vi "Action.vi"(7 "Assert Message":T1, 8 "error in (no error)":errorcluster, 11 "Pause Application in":refnum<class "Pause Application.lvclass">) -> (0 "error out":errorcluster)   [LabVIEW 2016, in "Assert API Components.lvlib" / "Log Assert Core.lvlib" / "Pause Application.lvclass"]
doc: "Dynamic dispatch vi which is triggered when an assert fails and the failure action is set to Pause.\nPauses the application and highlights the item which failed."
uses:
  Pause Application.lvclass
  Message Data.ctl
  Failure Actions.ctl
  VI References.ctl
  <vilib>/Utility/traverseref.llb/TRef TravTarget.ctl
  <vilib>/Utility/traverseref.llb/VI Scripting - Traverse.lvlib
  Assert API Components.lvlib
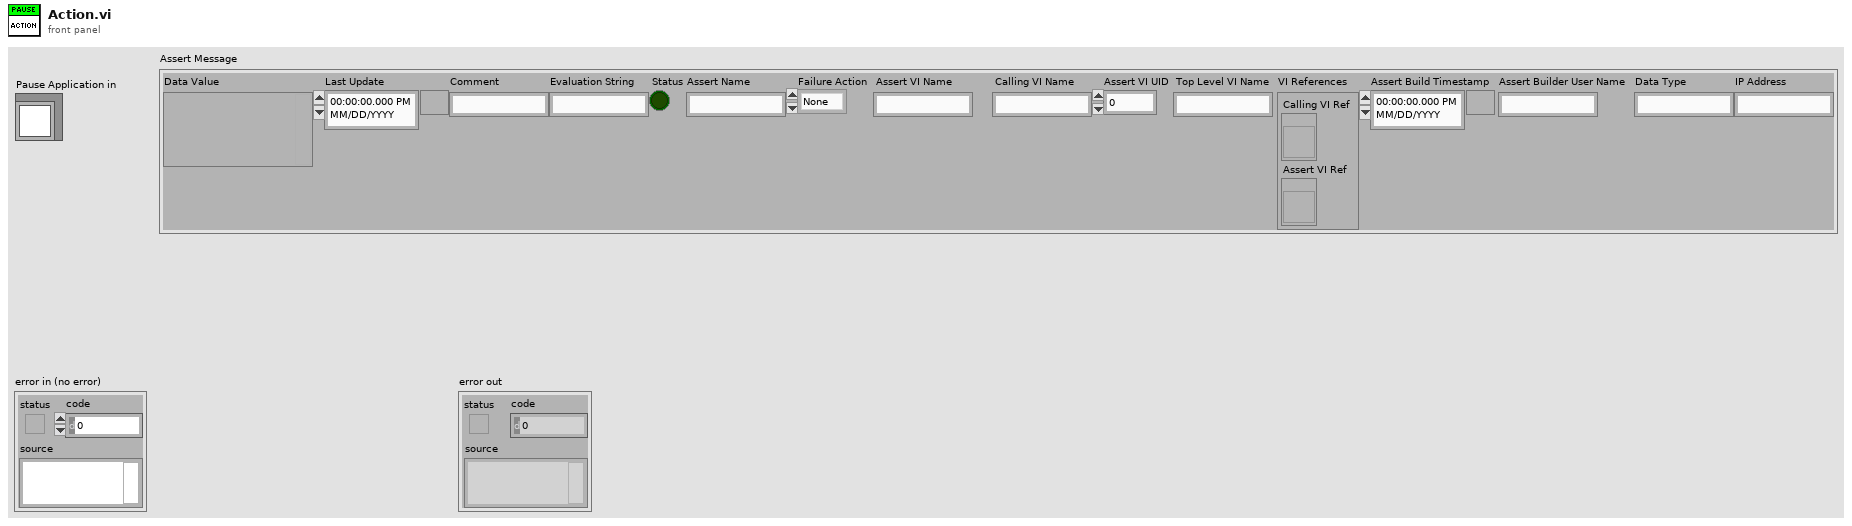
[diagram p1: front panel]
types:
  T1 = typedef "Assert API Components.lvlib/Message Data.ctl" = cluster{"Data Value":variant, "Last Update":timestamp, "Comment":string, "Evaluation String":string, "Status":bool, "Assert Name":string, "Failure Action":T2, "Assert VI Name":string, "Calling VI Name":string, "Assert VI UID":i32, "Top Level VI Name":string, "VI References":T3, "Assert Build Timestamp":timestamp, "Assert Builder User Name":string, "Data Type":string, "IP Address":string}
  T2 = typedef "Assert API Components.lvlib/Failure Actions.ctl" = enum16{"None", "Log To File", "Pause Execution", "Abort Execution"}
  T3 = typedef "Assert API Components.lvlib/VI References.ctl" = cluster{"Calling VI Ref":refnum<vi>, "Assert VI Ref":refnum<vi>}
  T4 = typedef "TRef TravTarget.ctl" = enum16{"FP", "BD", "Other"}
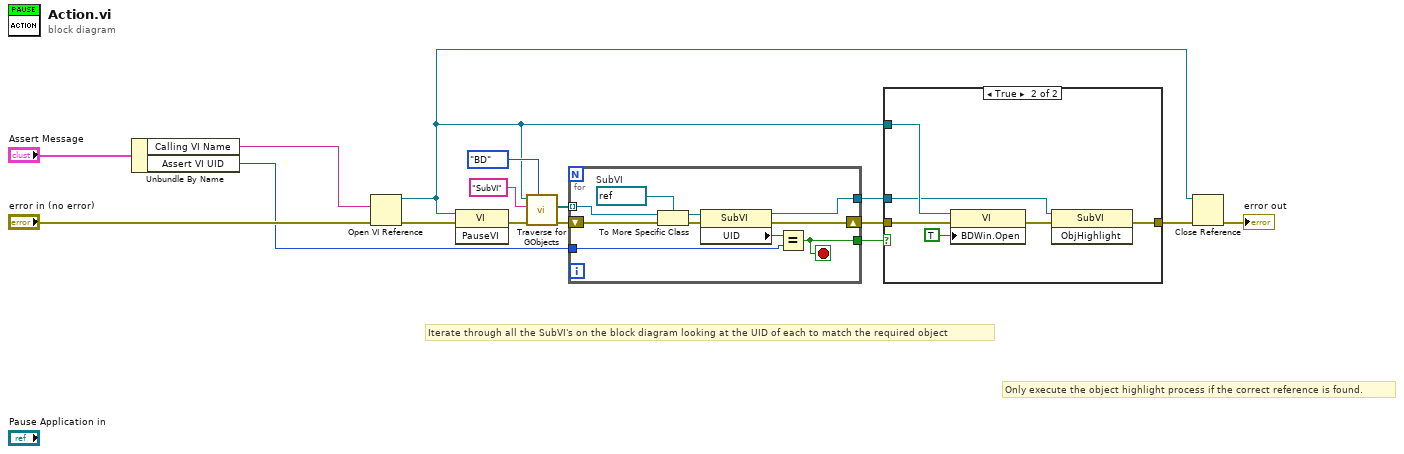
[diagram p0: block diagram]
diagram:
  # "Only execute the object highlight process if the correct reference is found."
  # "Iterate through all the SubVI's on the block diagram looking at the UID of each to match the required object"
  n1 = Unbundle By Name("Assert Message") -> ("Calling VI Name"=w3:string, "Assert VI UID"=w12:i32)
  n2 = Open VI Reference(vi path=w3, error in (no error)="error in (no error)") -> (vi reference=w1:refnum<vi>, error out=w4:errorcluster)  [unwired: 4 in]
  n3 = invoke class="VI" method="PauseVI"(reference=w1, error in=w4) -> (error out=w5:errorcluster)  [unwired: 1 in, 2 out]
  n4 = call <vilib>:"Traverse for GObjects.vi"("Traverse Target"=TRef_TravTarget."BD", "error in (no error)"=w5, "Class Name"="SubVI", "VI Refnum"=w1) -> ("error out"=w14:errorcluster, "References"=w15:refnum<vi>[])  [unwired: 4 in, 2 out]
  n5 = for {
    tunnel: w15 -> [w19] mode=indexing
    tunnel: w12 -> [w25]
    tunnel: [w24] -> w6
    tunnel: [w23] -> w9
    shift-right: [w22] -> w8
    shift-left: w14 -> [w21]
    stop <- w24 stop-if-true
    w17 = refnum<vi> refnum  # SubVI
    n6 = To More Specific Class(target class=w17, reference=w19, error in=w21) -> (specific class reference=w18:refnum<vi>, error out=w20:errorcluster)
    n7 = property class="SubVI"(reference=w18, error in=w20) -> (reference out=w23:refnum<vi>, error out=w22:errorcluster, "UID"=w26:i32)
    n8 = Equal?(x=w26, y=w25) -> (x = y?=w24:bool)
  }
  n9 = case shown="True" w6 {
    tunnel: w1 -> [_ w31]
    tunnel: w9 -> [_ w30]
    tunnel: w8 -> [w27 w29]
    tunnel: [w27 w28] -> w7
    frame False {
    }
    frame True {
      n10 = property class="VI"(reference=w31, error in=w29, "BDWin.Open"=TRUE ("Block Diagram Window:Open")) -> (error out=w33:errorcluster)  [unwired: 1 out]
      n11 = invoke class="SubVI" method="ObjHighlight"(reference=w30, error in=w33) -> (error out=w28:errorcluster)  [unwired: 1 in, 2 out]
    }
  }
  n12 = Close Reference(reference=w1, error in (no error)=w7) -> (error out=→"error out":errorcluster)
